vi "Rig_Pict_Display_Pref.vi"(0 "Traverse Name":string) -> (1 "Roll Pitch Yaw ADAM Channels":string[](array[string]), 4 "Which Axis is vertical?":enum16{"X Axis", "Y Axis", "Z Axis"}(ring), 6 "Plan View":T1, 7 "Side View":T1, 8 "Front View":T1)   [LabVIEW 2011]
uses:
  Pict_Plot_Axis.ctl
  Axis.ctl
  Globals/Constants_global.vi
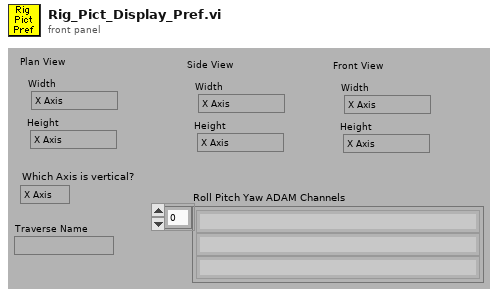
[diagram p1: front panel]
types:
  T1 = typedef "Pict_Plot_Axis.ctl" = cluster{"Width":T2, "Height":T2}
  T2 = typedef "Axis.ctl" = enum16{"X Axis", "X Axis -ve", "Y Axis", "Y Axis -ve", "Z Axis", "Z Axis -ve"}
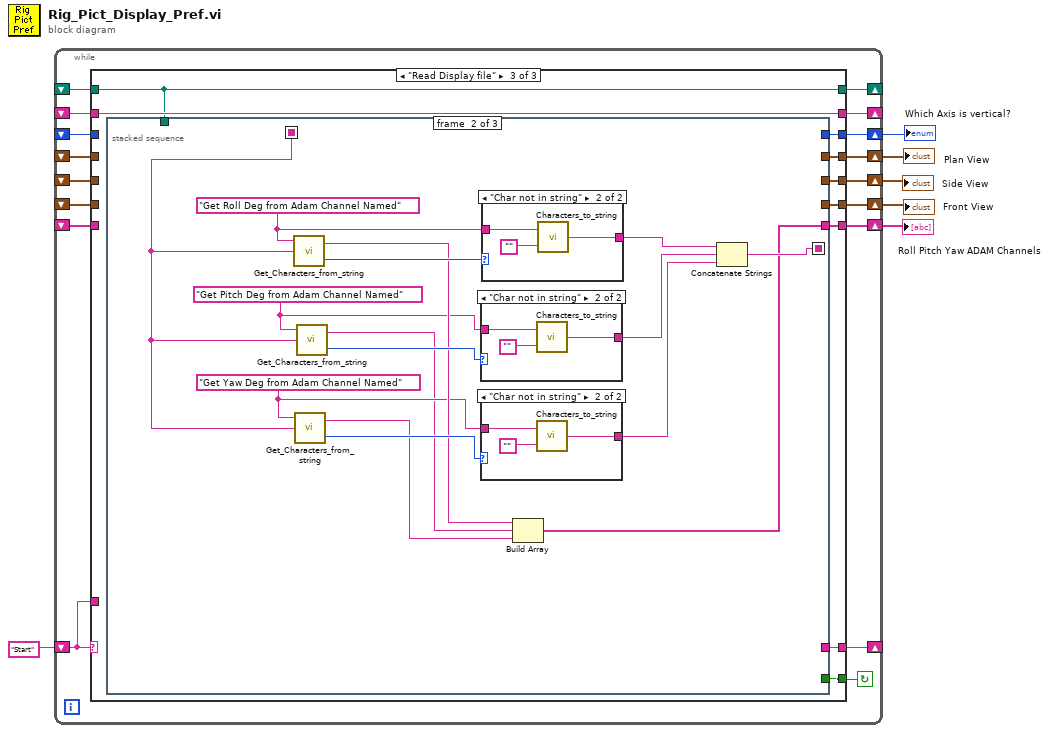
[diagram p0: block diagram]
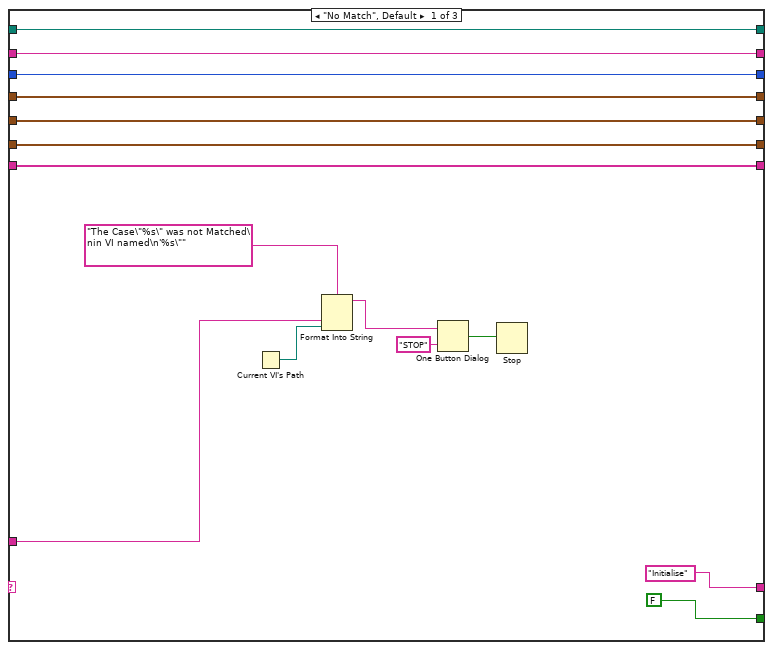
[diagram p2: hidden frame]
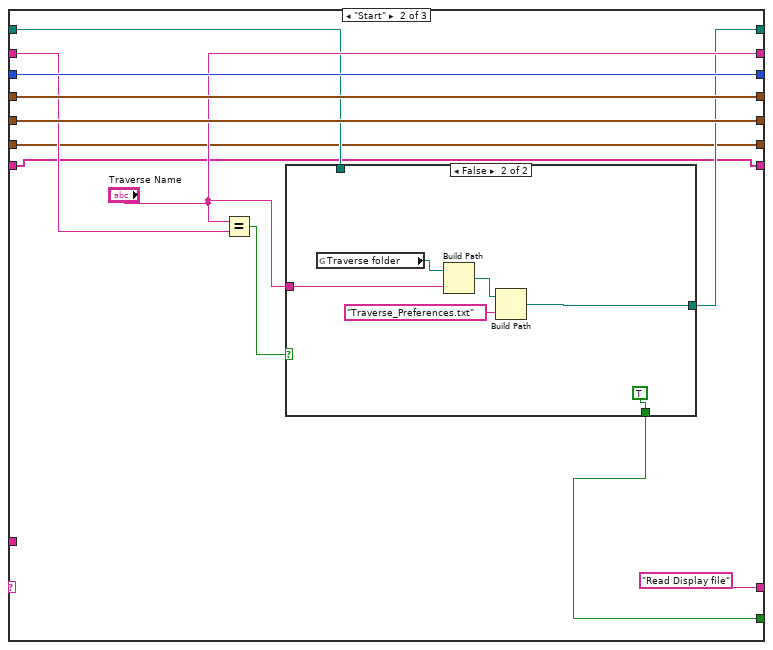
[diagram p3: hidden frame]
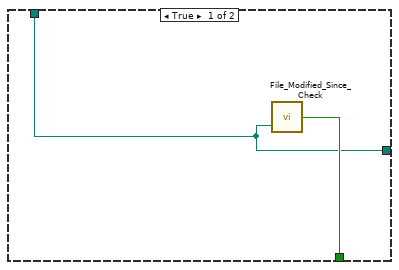
[diagram p4: hidden frame]
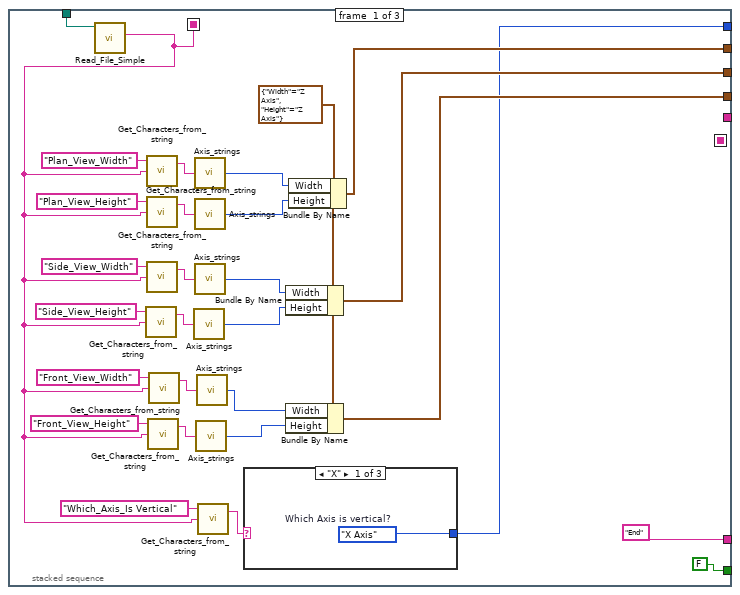
[diagram p5: hidden frame]
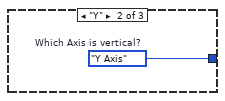
[diagram p6: hidden frame]
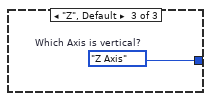
[diagram p7: hidden frame]
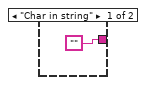
[diagram p8: hidden frame]
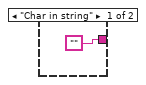
[diagram p9: hidden frame]
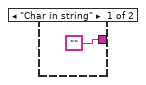
[diagram p10: hidden frame]
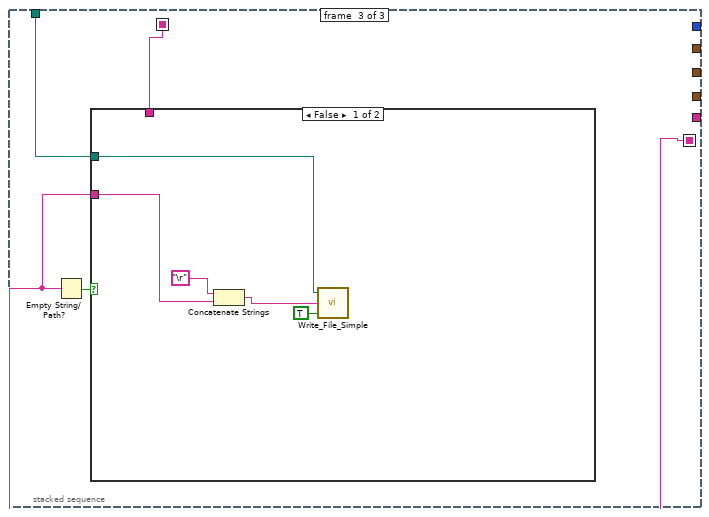
[diagram p11: hidden frame]
diagram:
  n1 = while {
    shift-left: "Start" -> [w21]
    shift-right: [w22] -> _
    shift-right: [w19] -> _
    shift-left: _ -> [w20]
    shift-right: [w13] -> w2
    shift-left: _ -> [w14]
    shift-right: [w16] -> w5
    shift-left: _ -> [w15]
    shift-right: [w17] -> w4
    shift-left: _ -> [w18]
    shift-right: [w12] -> _
    shift-left: _ -> [w11]
    shift-right: [w9] -> w3
    shift-left: _ -> [w10]
    shift-right: [w8] -> w1
    shift-left: _ -> [w7]
    stop <- w23 continue-if-true
    n2 = case shown="\"Read Display file\"" w21 {
      tunnel: [FALSE w43 w60] -> w23
      tunnel: ["Initialise" "Read Display file" w67] -> w22
      tunnel: w21 -> [w33 _ _]
      tunnel: w20 -> [w29 w46 w66]
      tunnel: [w29 "Traverse Name" w66] -> w19
      tunnel: w18 -> [w26 w49 _]
      tunnel: [w26 w49 w63] -> w17
      tunnel: [w27 w48 w64] -> w16
      tunnel: w15 -> [w27 w48 _]
      tunnel: w14 -> [w28 w47 _]
      tunnel: [w28 w47 w61] -> w13
      tunnel: [w30 w44 w65] -> w12
      tunnel: w11 -> [w30 w41 w65]
      tunnel: w10 -> [w25 w40 _]
      tunnel: [w25 w40 w62] -> w9
      tunnel: [w24 w39 w59] -> w8
      tunnel: w7 -> [w24 w39 _]
      frame "No Match", Default {
        n3 = Current VI's Path() -> (path=w32:path)
        n4 = Format Into String(format string="The Case\"%s\" was not Matched\nin VI named\n'%s\"" ("Format String"), w33, w32) -> (resulting string=w36:string)  [unwired: 2 in, 1 out]
        n5 = One Button Dialog(message=w36, button name ("OK")="STOP") -> (true=w34:bool)
        n6 = Stop(stop? (T)=w34) -> ()
      }
      frame "Start" {
        n7 = Equal?(x="Traverse Name", y=w46) -> (x = y?=w42:bool)
        n8 = case shown="False" w42 {
          tunnel: "Traverse Name" -> [_ w57]
          tunnel: [w51 w54] -> w44
          tunnel: [w52 TRUE ("Modified?")] -> w43
          tunnel: w41 -> [w51 _]
          frame True {
            n9 = call "File_Modified_Since_Check.vi"("Pathname"=w51) -> ("Modified?"=w52:bool)  [unwired: 1 in]
          }
          frame False {
            n10 = global read "Constants_global.vi" "Traverse folder"() -> (w58:path)
            n11 = Build Path(base path=w58, name or relative path=w57) -> (appended path=w56:path)
            n12 = Build Path(base path=w56, name or relative path="Traverse_Preferences.txt") -> (appended path=w54:path)
          }
        }
      }
      frame "Read Display file" {
        n13 = stacked-sequence {
          seq-local: [w68 _ _] -> [_ w114 w129]
          seq-local: [_ w101 _] -> [_ _ w128]
          tunnel: ["End" _ _] -> w67
          tunnel: w65 -> [w95 _ w127]
          tunnel: [w75 _ _] -> w64
          tunnel: [w74 _ _] -> w63
          tunnel: [w73 _ _] -> w62
          tunnel: [w70 _ _] -> w61
          tunnel: [FALSE ("Modified?") _ _] -> w60
          tunnel: [_ w100 _] -> w59
          frame #0 {
            w80 = T1 {"Width"=enum."Z Axis", "Height"=enum."Z Axis"} ("Plot Axis")
            n14 = call "Read_File_Simple.vi"("Filename"=w95) -> ("string"=w68:string)  [unwired: 2 in, 7 out]
            n15 = call "Get_Characters_from_string.vi"("Input string"=w68, "Variable name"="Side_View_Height") -> ("Value"=w88:string)  [unwired: 1 in, 1 out]
            n16 = call "Get_Characters_from_string.vi"("Input string"=w68, "Variable name"="Plan_View_Width") -> ("Value"=w93:string)  [unwired: 1 in, 1 out]
            n17 = call "Get_Characters_from_string.vi"("Input string"=w68, "Variable name"="Plan_View_Height") -> ("Value"=w92:string)  [unwired: 1 in, 1 out]
            n18 = call "Get_Characters_from_string.vi"("Input string"=w68, "Variable name"="Side_View_Width") -> ("Value"=w89:string)  [unwired: 1 in, 1 out]
            n19 = call "Get_Characters_from_string.vi"("Input string"=w68, "Variable name"="Front_View_Height") -> ("Value"=w84:string)  [unwired: 1 in, 1 out]
            n20 = call "Get_Characters_from_string.vi"("Input string"=w68, "Variable name"="Front_View_Width") -> ("Value"=w85:string)  [unwired: 1 in, 1 out]
            n21 = call "Axis_strings.vi"("String"=w88) -> ("Enum"=w76:T2)
            n22 = call "Axis_strings.vi"("String"=w93) -> ("Enum"=w79:T2)
            n23 = call "Axis_strings.vi"("String"=w92) -> ("Enum"=w78:T2)
            n24 = call "Axis_strings.vi"("String"=w89) -> ("Enum"=w77:T2)
            n25 = call "Axis_strings.vi"("String"=w84) -> ("Enum"=w81:T2)
            n26 = call "Axis_strings.vi"("String"=w85) -> ("Enum"=w82:T2)
            n27 = call "Get_Characters_from_string.vi"("Input string"=w68, "Variable name"="Which_Axis_Is Vertical") -> ("Value"=w71:string)  [unwired: 1 in, 1 out]
            n28 = case shown="\"X\"" w71 {
              tunnel: [w97 w98 w99] -> w70
              frame "X" {
                w97 = enum16{"X Axis", "Y Axis", "Z Axis"}."X Axis"  # Which Axis is vertical?
              }
              frame "Y" {
                w98 = enum16{"X Axis", "Y Axis", "Z Axis"}."Y Axis"  # Which Axis is vertical?
              }
              frame "Z", Default {
                w99 = enum16{"X Axis", "Y Axis", "Z Axis"}."Z Axis"  # Which Axis is vertical?
              }
            }
            n29 = Bundle By Name(cluster=w80, "Width"=w77, "Height"=w76) -> (w74:T1)
            n30 = Bundle By Name(cluster=w80, "Width"=w82, "Height"=w81) -> (w73:T1)
            n31 = Bundle By Name(cluster=w80, "Width"=w79, "Height"=w78) -> (w75:T1)
          }
          frame #1 {
            w104 = "Get Yaw Deg from Adam Channel Named" ("Variable name")
            w105 = "Get Pitch Deg from Adam Channel Named" ("Variable name")
            w112 = "Get Roll Deg from Adam Channel Named" ("Variable name")
            n32 = call "Get_Characters_from_string.vi"("Input string"=w114, "Variable name"=w112) -> ("Status"=w113:enum16{"Char in string", "Char not in string"}, "Value"=w106:string)  [unwired: 1 in]
            n33 = call "Get_Characters_from_string.vi"("Input string"=w114, "Variable name"=w104) -> ("Status"=w109:enum16{"Char in string", "Char not in string"}, "Value"=w102:string)  [unwired: 1 in]
            n34 = call "Get_Characters_from_string.vi"("Input string"=w114, "Variable name"=w105) -> ("Status"=w110:enum16{"Char in string", "Char not in string"}, "Value"=w103:string)  [unwired: 1 in]
            n35 = case shown="\"Char not in string\"" w110 {
              tunnel: w105 -> [_ w122]
              tunnel: ["" w120] -> w108
              frame "Char in string" {
              }
              frame "Char not in string" {
                n36 = call "Characters_to_string.vi"("Characters to write"="", "Label for characters"=w122) -> ("Output string"=w120:string)
              }
            }
            n37 = case shown="\"Char not in string\"" w109 {
              tunnel: w104 -> [_ w118]
              tunnel: ["" w116] -> w107
              frame "Char in string" {
              }
              frame "Char not in string" {
                n38 = call "Characters_to_string.vi"("Characters to write"="", "Label for characters"=w118) -> ("Output string"=w116:string)
              }
            }
            n39 = case shown="\"Char not in string\"" w113 {
              tunnel: w112 -> [_ w126]
              tunnel: ["" w124] -> w111
              frame "Char in string" {
              }
              frame "Char not in string" {
                n40 = call "Characters_to_string.vi"("Characters to write"="", "Label for characters"=w126) -> ("Output string"=w124:string)
              }
            }
            n41 = Build Array(w106, w103, w102) -> (w100:string[])
            n42 = Concatenate Strings(w111, w108, w107) -> (w101:string)
          }
          frame #2 {
            n43 = Empty String/Path?(string/path=w128) -> (empty?=w130:bool)
            n44 = case shown="False" w130 {
              tunnel: w129 -> [_ _]
              tunnel: w128 -> [w132 _]
              tunnel: w127 -> [w135 _]
              frame False {
                n45 = Concatenate Strings("\r", w132) -> (w131:string)
                n46 = call "Write_File_Simple.vi"("append to file? (new file:F)"=TRUE, "character string"=w131, "file path"=w135) -> ()  [unwired: 2 out]
              }
              frame True {
              }
            }
          }
        }
      }
    }
  }
  "Plan View" <- w5
  "Side View" <- w4
  "Front View" <- w3
  "Which Axis is vertical?" <- w2
  "Roll Pitch Yaw ADAM Channels" <- w1
